vi "DVR.vars.Read.vi"(8 "error in":errorcluster, 11 "DVR.state":T3) -> (0 "error out":errorcluster, 2 "vars":T1={"save"={"base_folder"={"Folder"=path "", "tif"=FALSE, "jpg"=FALSE}, "module"="", "#"=20, "sub#"=0, "save.op"=enum."Full", "same?"=FALSE, "Shift"=enum."Single", "jpg?"=FALSE, "flip"={"x"=FALSE, "y"=FALSE}}, "acq"={"# Acq"=100, "rotate"=FALSE, "FPS"=0.0}, "calib.manual"={"BG"={"Image"=[], "enabled?"=FALSE}, "FF"={"Image"=[], "enabled?"=FALSE}}})   [LabVIEW 2020]
uses:
  _controls/data.ctl
  camera/camera.lvclass
  _controls/data.ref.ctl
  <vilib>/vision/Image Controls.llb/IMAQ Image.ctl
  _controls/state.ctl
  _controls/data.vars.ctl
  _controls/flip.ctl
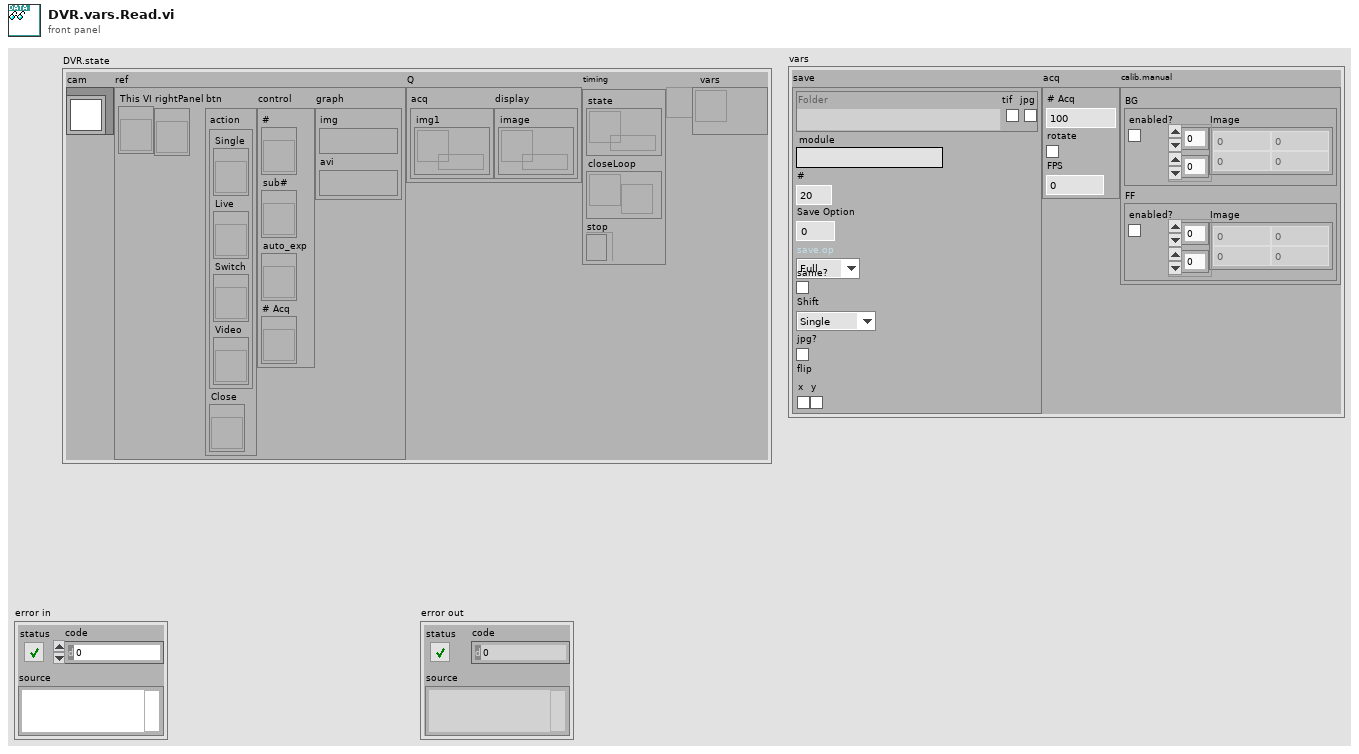
[diagram p1: front panel]
types:
  T1 = typedef "data.vars.ctl" = cluster{"save":cluster{"base_folder":cluster{"Folder":path, "tif":bool, "jpg":bool}, "module":string, "#":u32, "sub#":u8, "save.op":enum16{"Full", "Light"}, "same?":bool, "Shift":enum16{"Single", "Leapfrog"}, "jpg?":bool, "flip":T2}, "acq":cluster{"# Acq":u16, "rotate":bool, "FPS":dbl}, "calib.manual":cluster{"BG":cluster{"Image":u16[][], "enabled?":bool}, "FF":cluster{"Image":u16[][], "enabled?":bool}}}
  T2 = typedef "flip.ctl" = cluster{"x":bool, "y":bool}
  T3 = typedef "data.ctl" = cluster{"cam":refnum<class "camera.lvclass">, "ref":T4, "Q":cluster{"acq":cluster{"img1":refnum<queue>}, "display":cluster{"image":refnum<queue>}}, "timing":cluster{"state":refnum<queue>, "closeLoop":refnum<notifier>, "stop":refnum<k4>}, "vars":refnum<data-value>}
  T4 = typedef "data.ref.ctl" = cluster{"This VI":refnum<vi>, "rightPanel":refnum<vi>, "btn":cluster{"action":cluster{"Single":refnum<vi>, "Live":refnum<vi>, "Switch":refnum<vi>, "Video":refnum<vi>}, "Close":refnum<vi>}, "control":cluster{"#":refnum<vi>, "sub#":refnum<vi>, "auto_exp":refnum<vi>, "# Acq":refnum<vi>}, "graph":cluster{"img":T5, "avi":T5}}
  T5 = typedef "IMAQ Image.ctl" = refnum<image>
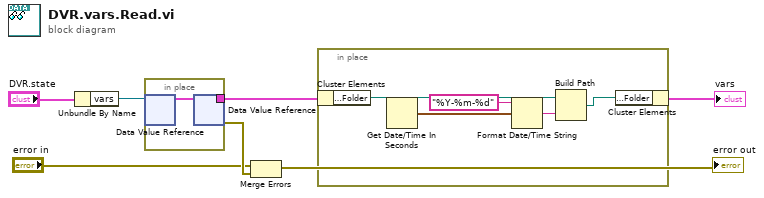
[diagram p0: block diagram]
diagram:
  n1 = Unbundle By Name("DVR.state") -> ("vars"=w3:refnum<data-value>)
  n2 = in-place {
    in-place-border: [w8] -> w2
    n3 = in-place-dvr #1(w3) -> (w8:T1)  [unwired: 1 out]
    n4 = in-place-dvr #1(w8) -> (w6:errorcluster)  [unwired: 1 out]
  }
  n5 = Merge Errors("error in", w6) -> (→"error out":errorcluster)
  n6 = in-place {
    n7 = in-place-cluster #2(w2) -> ("save.base_folder.Folder"=w10:path)
    n8 = Get Date/Time In Seconds() -> (seconds since 1Jan1904=w12:timestamp)
    n9 = Format Date/Time String(time format string (%c)="%Y-%m-%d", seconds (now)=w12) -> (date/time string=w13:string)  [unwired: 1 in]
    n10 = Build Path(base path=w10, name or relative path=w13) -> (appended path=w9:path)
    n11 = in-place-cluster #2("save.base_folder.Folder"=w9) -> (→"vars":T1)
  }
